vi "EXAMPLE_2.vi"() -> ()   [LabVIEW 2017]
uses:
  ZBOX_IS.lvlib
  <vilib>/Analysis/NI_AALBase.lvlib
  <vilib>/Analysis/baseanly.llb/Mean (DBL).vi
panel:
  in  "Get configuration data":bool
  in  "load comp":bool
  in  "load shunt":bool
  in  "Device Configuration File":path=path "SELECT Device Configuration File"
  out "Level":T1={"Slide 5"={1482, 2181}, "max OL 10"=FALSE, "max OL 9"=FALSE, "Slide 4"={1477, 2189}, "max OL 8"=FALSE, "max OL 7"=FALSE} {"Slide 4" scale=0.0..4096.0; "Slide 5" scale=0.0..4096.0}
  out "Application":string="EXAMPLE_3_1.vi"
  out "Battery Status":dbl
  out "Battery Voltage":dbl
  in  "DATA STREAMING":bool=TRUE
  out "writing":bool
  in  "Datalog file":string="Datalog_file_1.txt"
  out "CompValues":string="1000000000.00,1000000000.00,1000000000.00,1000000000.00,1000000000.00,1000000000.00,1000000000.00,1000000000.00,1000000000.00,1000000000.00,1000000000.00,1000000000.00,1000000000.00,1000000000.00,1000000000.00,       0.00,       0.00,       0.00,       0.00,       0.00,       0.00,       0.00,       0.00,       0.00,       0.00,       0.00,       0.00,       0.00,       0.00,       0.00"
  out "Shunt":string="     999.93,     999.93,     999.93,     999.93,     999.93,     999.93,     999.93,     999.93,     999.93,     999.93,     999.93,     999.93,     999.93,     999.92,     999.91,      -0.02,      -0.03,      -0.05,      -0.11,      -0.17,      -0.26,      -0.35,      -0.47,      -0.65,      -0.92,      -1.34,      -1.91,      -2.70,      -3.78,      -5.26"
  out "Frequencies":string="    1000.00Hz,    2000.00Hz,    3000.00Hz,    7000.00Hz,   11000.00Hz,   17000.00Hz,   23000.00Hz,   31000.00Hz,   43000.00Hz,   61000.00Hz,   89000.00Hz,  127000.00Hz,  179000.00Hz,  251000.00Hz,  349000.00Hz"
  in  "SAVE":bool
  out "Front End":string
  out "frequencies":dbl[](array[numeric])=[1000.0, 2000.0, 3000.0, 7000.0, 11000.0, 17000.0, 23000.0, 31000.0, 43000.0, 61000.0, 89000.0, 127000.0, 179000.0, 251000.0, 349000.0]
  out "DEVICE":bool
  out "Device":string
  in  "Ext_Trigger":bool
  in  "EN COMP":bool
  in  "MEAS COMP":bool
  in  "G2":u8(slide) scale=0.0..3.0
  in  "G1":u8(slide) scale=0.0..3.0
  out "Magnitude,   ohm":cluster{"freqs":dbl[], dbl[]}(graph)={"freqs"=[1000.0, 2000.0, 3000.0, 7000.0, 11000.0, 17000.0, 23000.0, 31000.0, 43000.0, 61000.0, 89000.0, 127000.0, 179000.0, 251000.0, 349000.0], [996.1091027832031, 996.1116979980469, 996.0496057128906, 996.1361779785157, 996.0625866699219, 996.056845703125, 996.0880285644531, 996.0972033691406, 996.0096704101562, 996.0107141113281, 995.8494006347656, 995.4951928710938, 994.7552624511719, 993.43984375, 991.5672961425781]}
  out "Phase, deg":cluster{"freqs":dbl[], dbl[]}(graph)={"freqs"=[1000.0, 2000.0, 3000.0, 7000.0, 11000.0, 17000.0, 23000.0, 31000.0, 43000.0, 61000.0, 89000.0, 127000.0, 179000.0, 251000.0, 349000.0], [-0.002247831257991493, -0.002652753913716879, -0.005691929007298313, -0.012889227512059733, -0.021220838949084282, -0.02892146535217762, -0.03975417457520962, -0.055281588807702065, -0.07622284047305584, -0.10836573675274849, -0.1603422838449478, -0.22576678663492203, -0.3038424688577652, -0.3925769108533859, -0.4546267157793045]}
  out "Connected":bool
  out "DFTBins":u16[](array[numeric])=[1, 2, 3, 7, 11, 17, 23, 31, 43, 61, 89, 127, 179, 251, 349]
  out "Status":string
  in  "Power Source":bool
  in  "Signal":u32(slide)=46 scale=0.0..100.0
  in  "Sample Rate Divider":u32(ring)=1 items=["1"=1, "2"=2, "4"=4, "6"=6, "8"=8, "10"=10, "12"=12, "14"=14, "16"=16, "20"=20, "24"=24, "28"=28, "32"=32, "40"=40, "48"=48, "56"=56, "64"=64, "80"=80, "96"=96, "112"=112, "128"=128, "160"=160, "192"=192, "196"=196, "224"=224, "256"=256, "320"=320, "384"=384, "448"=448, "512"=512, "640"=640, "768"=768, "896"=896, "1024"=1024, "1280"=1280, "1536"=1536, "1792"=1792]
  in  "stop":bool
  in  "# of packages":u32=50 min=1 step=1
  # "10"
  # "5"
  # "2"
  # "1"
  # "10"
  # "5"
  # "2"
  # "1"
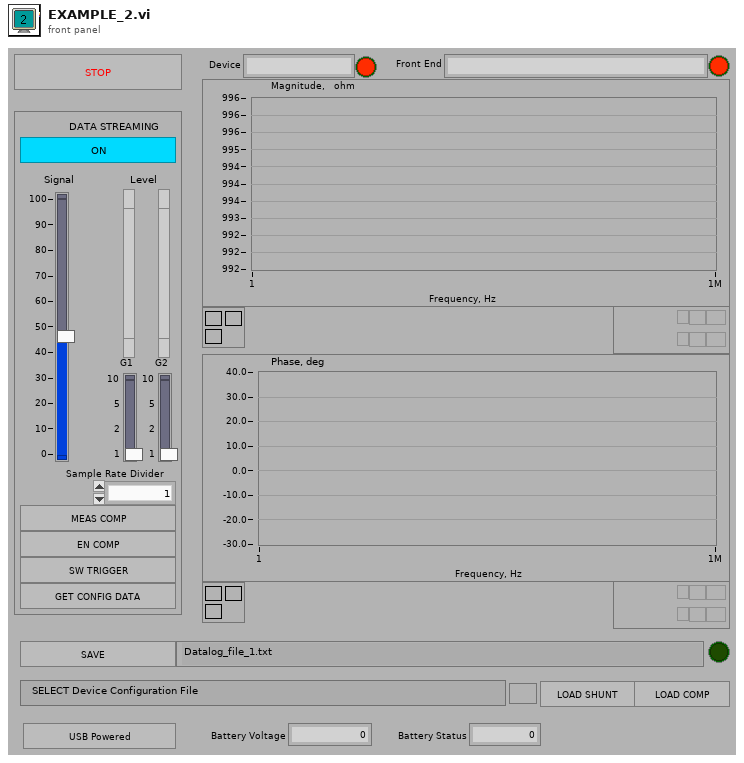
[diagram p1: front panel]
types:
  T1 = cluster{"Slide 5":cluster{u16, u16}, "max OL 10":bool, "max OL 9":bool, "Slide 4":cluster{u16, u16}, "max OL 8":bool, "max OL 7":bool}
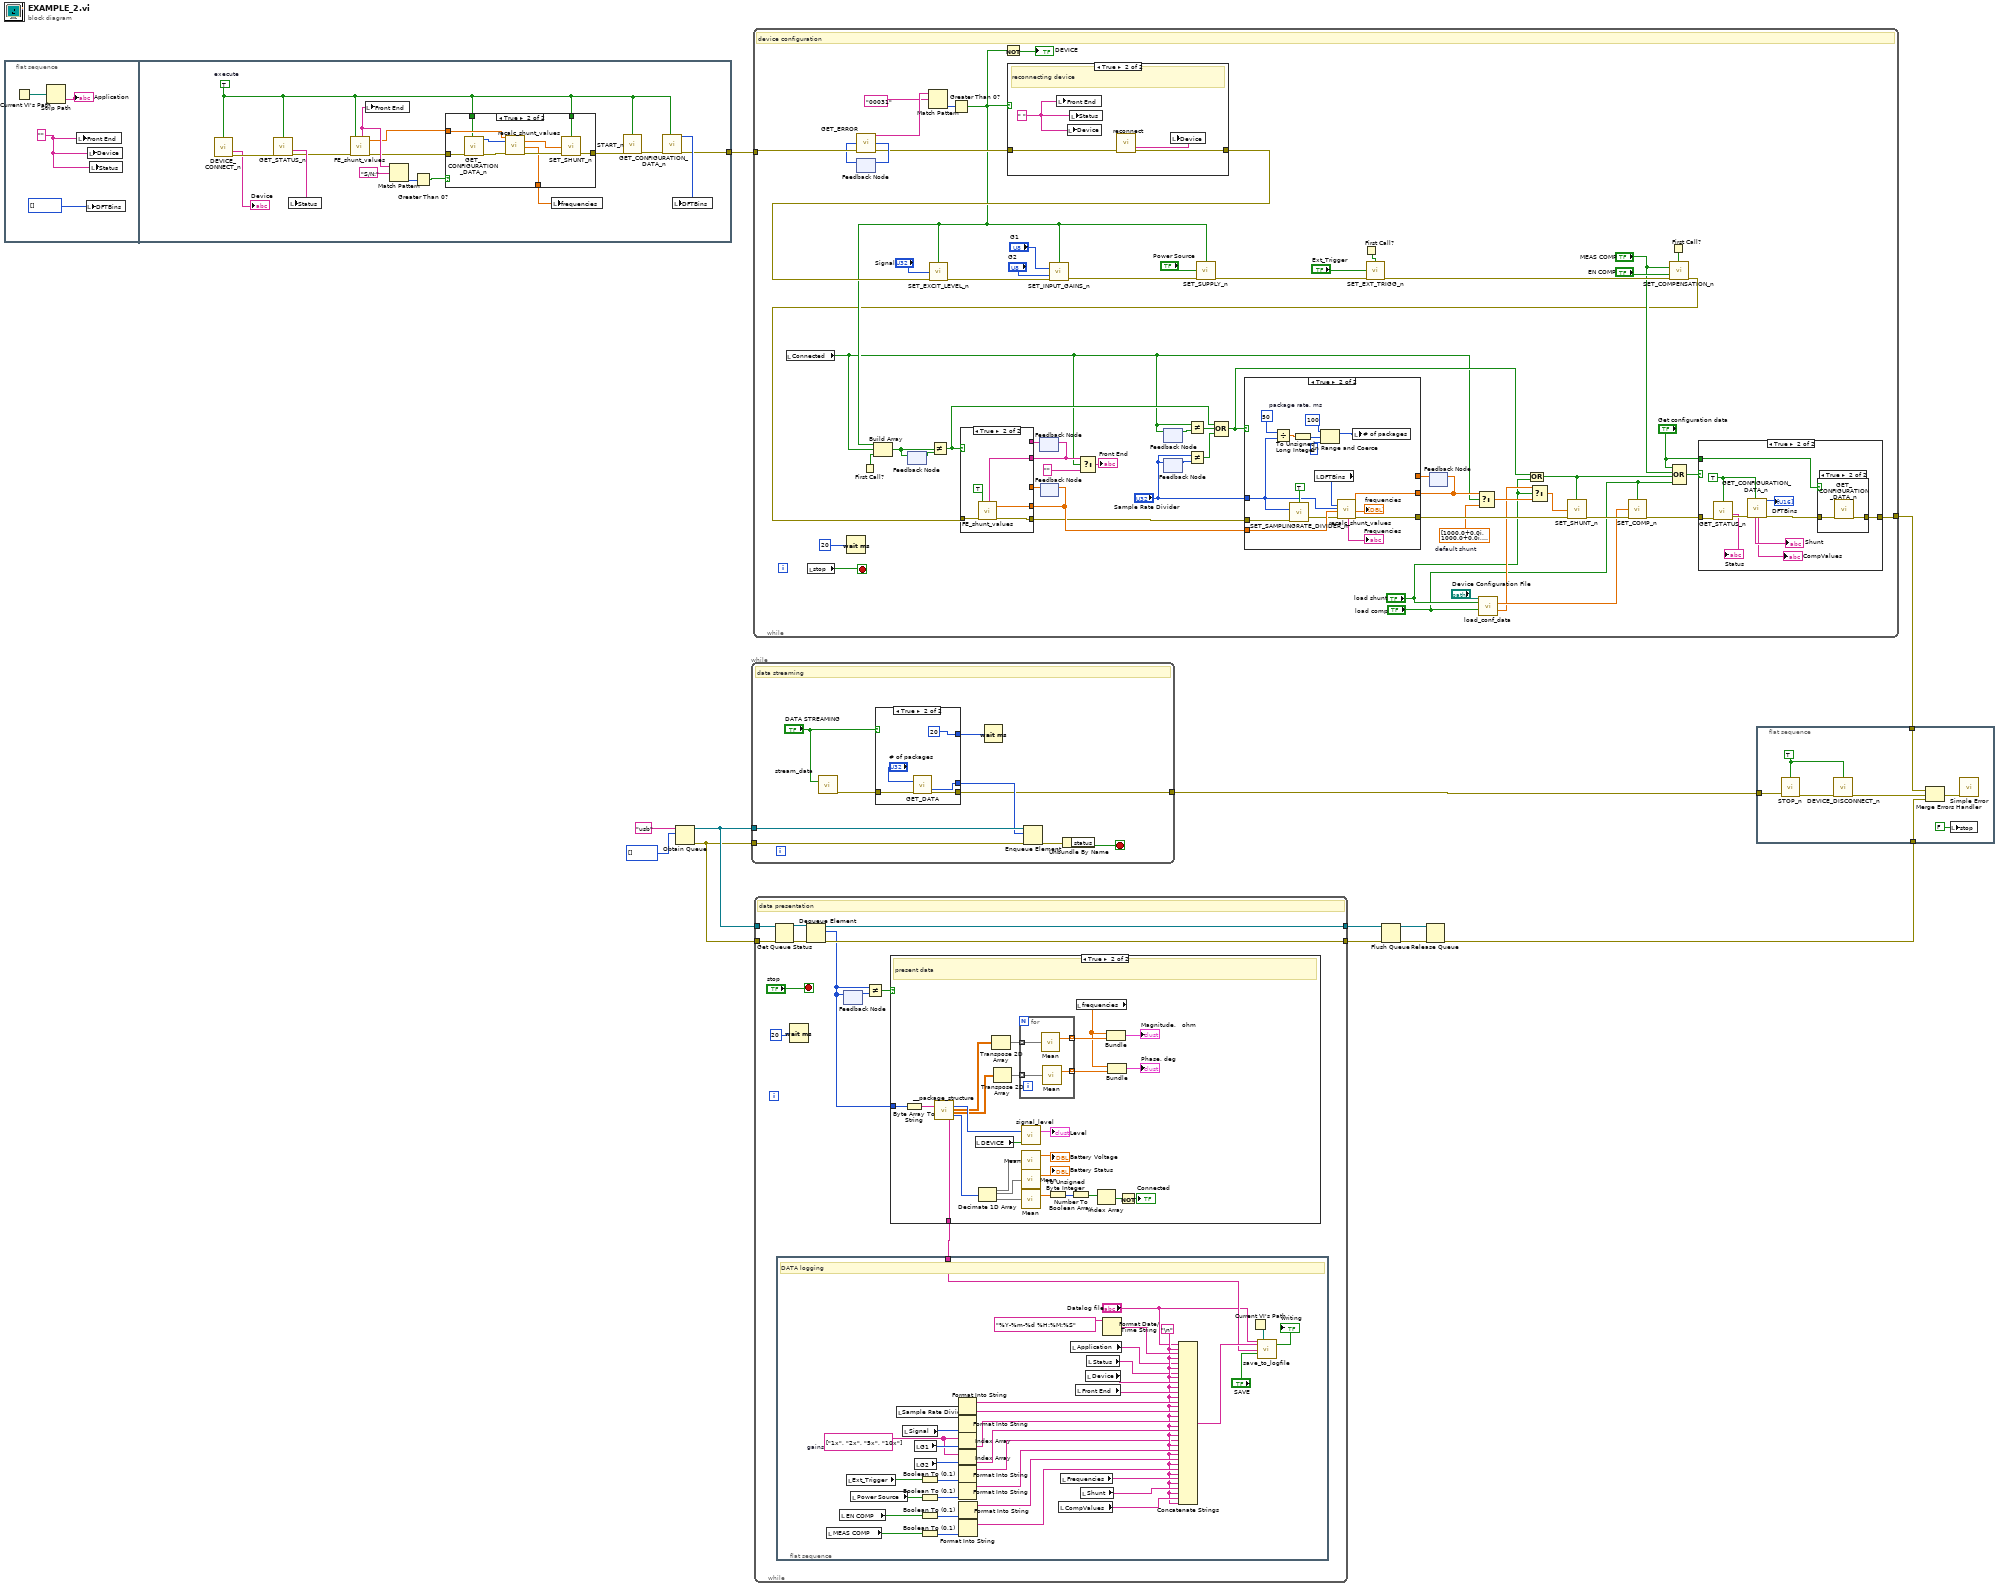
[diagram p0: block diagram]
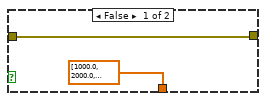
[diagram p2: hidden frame]
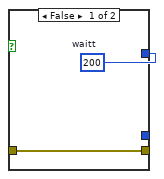
[diagram p3: hidden frame]
diagram:
  n1 = flat-sequence {
    tunnel: [w18] -> w7
    frame #0 {
      w16 = "" ("function return 2")
      n2 = Current VI's Path() -> (path=w13:path)
      n3 = Strip Path(path=w13) -> (name=→"Application":string)  [unwired: 1 out]
      n4 = local write "Front End"(w16) -> ()
      n5 = local write "DFTBins"(i32[] [] ("DFTBins")) -> ()
      n6 = local write "Device"(w16) -> ()
      n7 = local write "Status"(w16) -> ()
    }
    frame #1 {
      w17 = TRUE  # execute
      n8 = call "DEVICE_CONNECT_n.vi"("execute"=w17) -> ("serial no"=→"Device":string, "error out"=w32:errorcluster)  [unwired: 11 in, 2 out]
      n9 = call "GET_STATUS_n.vi"("execute"=w17, "error in (no error)"=w32) -> ("serial no"=w30:string, "error out"=w22:errorcluster)  [unwired: 10 in, 2 out]
      n10 = local write "Status"(w30) -> ()
      n11 = call "FE_shunt_values.vi"("error in (no error)"=w22, "execute"=w17) -> ("shunt"=w28:string, "FE_shunt_data"=w23:sgl[], "error out"=w24:errorcluster)  [unwired: 14 in, 1 out]
      n12 = local write "Front End"(w28) -> ()
      n13 = Match Pattern(string=w28, regular expression="S/N:") -> (offset past match=w26:i32)  [unwired: 1 in, 3 out]
      n14 = Greater Than 0?(x=w26) -> (x > 0?=w29:bool)
      n15 = case shown="True" w29 {
        tunnel: w23 -> [_ w44]
        tunnel: w24 -> [w33 w41]
        tunnel: [dbl[] [1000.0, 2000.0, 3000.0, 7000.0, 11000.0, 17000.0, 23000.0, 31000.0, 43000.0, 61000.0, 89000.0, 127000.0, 179000.0, 251000.0, 349000.0] ("freqs") w38] -> w25
        tunnel: [w33 w37] -> w21
        tunnel: w17 -> [_ w36]
        tunnel: w17 -> [_ w35]
        frame False {
        }
        frame True {
          n16 = call "GET_CONFIGURATION_DATA_n.vi"("error in (no error)"=w41, "execute"=w36) -> ("DFTBins"=w39:u16[], "error out"=w40:errorcluster)  [unwired: 7 in, 9 out]
          n17 = call "recalc_shunt_values.vi"("DFTBins"=w39, "FE_shunt_data"=w44, "error in (no error)"=w40) -> ("shunt"=w42:cdb[], "freqs"=w38:dbl[], "error out"=w43:errorcluster)  [unwired: 13 in, 1 out]
          n18 = call "SET_SHUNT_n.vi"("execute"=w35, "SHUNT values"=w42, "error in (no error)"=w43) -> ("error out"=w37:errorcluster)  [unwired: 11 in, 1 out]
        }
      }
      n19 = local write "frequencies"(w25) -> ()
      n20 = call "START_n.vi"("execute"=w17, "error in (no error)"=w21) -> ("error out"=w19:errorcluster)  [unwired: 12 in, 1 out]
      n21 = call "GET_CONFIGURATION_DATA_n.vi"("error in (no error)"=w19, "execute"=w17) -> ("DFTBins"=w20:u16[], "error out"=w18:errorcluster)  [unwired: 7 in, 9 out]
      n22 = local write "DFTBins"(w20) -> ()
    }
  }
  n23 = Obtain Queue(name (unnamed)="usb", element data type=u8[] [] ("unsigned byte array 2")) -> (queue out=w9:refnum<queue>, error out=w8:errorcluster)  [unwired: 3 in, 1 out]
  n24 = while {
    tunnel: w9 -> [w53]
    tunnel: w8 -> [w52]
    tunnel: [w46] -> w6
    stop <- w51 stop-if-true
    # "data streaming"
    n25 = call "stream_data.vi"("DATA STREAMING"="DATA STREAMING") -> ("error out"=w49:errorcluster)  [unwired: 14 in]
    n26 = case shown="True" "DATA STREAMING" {
      tunnel: [_ w60] -> w47
      tunnel: [w54 u32 20 ("wait")] -> w50
      tunnel: w49 -> [w55 w59]
      tunnel: [w55 w58] -> w46
      frame False {
        w54 = u32 200  # waitt
      }
      frame True {
        n27 = call "GET_DATA.vi"("ulValue"="# of packages", "error in (no error)"=w59) -> ("BytePtr"=w60:u8[], "error out"=w58:errorcluster)  [unwired: 11 in, 1 out]
      }
    }
    n28 = Wait (ms)(milliseconds to wait=w50) -> ()  [unwired: 1 out]
    n29 = Enqueue Element(queue=w53, element=w47, error in (no error)=w52) -> (error out=w45:errorcluster)  [unwired: 3 out]
    n30 = Unbundle By Name(w45) -> ("status"=w51:bool)
  }
  n31 = while {
    tunnel: w7 -> [w109]
    tunnel: [w71] -> w4
    stop <- w61 stop-if-true
    w94 = cdb[] [1000.0+0.0i, 1000.0+0.0i, 1000.0+0.0i, 1000.0+0.0i, 1000.0+0.0i, 1000.0+0.0i, 1000.0+0.0i, 1000.0+0.0i, 1000.0+0.0i, 1000.0+0.0i, 1000.0+0.0i, 1000.0+0.0i, 1000.0+0.0i, 1000.0+0.0i, 1000.0+0.0i]  # default shunt
    # "device configuration"
    n32 = local read "Connected"() -> (w78:bool)
    n33 = local read "stop"() -> (w61:bool)
    n34 = Wait (ms)(milliseconds to wait=u32 20 ("wait")) -> ()  [unwired: 1 out]
    n35 = feedback #1() -> (w106:u32[])  [unwired: 1 in]
    n36 = call "GET_ERROR.vi"("uLPtr"=w106, "error in (no error)"=w109) -> ("function return"=w105:string, "uLPtr"=w107:u32[], "error out"=w103:errorcluster)  [unwired: 11 in]
    n37 = feedback-in #1(w107) -> ()
    n38 = First Call?() -> (First Call?: T/F=w98:bool)
    n39 = feedback #2() -> (w93:bool[])  [unwired: 1 in]
    n40 = Match Pattern(string=w105, regular expression="00031" ("substring 2")) -> (offset past match=w108:i32)  [unwired: 1 in, 3 out]
    n41 = Greater Than 0?(x=w108) -> (x > 0?=w83:bool)
    n42 = Build Array(w83, w78, w98) -> (w92:bool[])
    n43 = feedback-in #2(w92) -> ()
    n44 = Not Equal?(x=w92, y=w93) -> (x != y?=w79:bool)
    n45 = Not(x=w83) -> (.not. x?=→"DEVICE":bool)
    n46 = case shown="True" w83 {
      tunnel: w103 -> [w122 w126]
      tunnel: [w122 w125] -> w97
      frame False {
      }
      frame True {
        w123 = " " ("status")
        # "reconnecting device"
        n47 = local write "Front End"(w123) -> ()
        n48 = local write "Device"(w123) -> ()
        n49 = local write "Status"(w123) -> ()
        n50 = call "reconnect.vi"("error in (no error)"=w126) -> ("serial no"=w124:string, "error out"=w125:errorcluster)  [unwired: 12 in, 1 out]
        n51 = local write "Device"(w124) -> ()
      }
    }
    n52 = call "SET_EXCIT_LEVEL_n.vi"("execute"=w83, "Level"="Signal", "error in (no error)"=w97) -> ("error out"=w117:errorcluster)  [unwired: 11 in, 1 out]
    n53 = feedback #3() -> (w115:string)  [unwired: 1 in]
    n54 = feedback #4() -> (w116:sgl[])  [unwired: 1 in]
    n55 = call "SET_INPUT_GAINS_n.vi"("execute"=w83, "G1"="G1", "G2"="G2", "error in (no error)"=w117) -> ("error out"=w110:errorcluster)  [unwired: 10 in, 1 out]
    n56 = feedback #5() -> (w91:bool)  [unwired: 1 in]
    n57 = feedback-in #5(w78) -> ()
    n58 = feedback #6() -> (w90:u32)  [unwired: 1 in]
    n59 = feedback-in #6("Sample Rate Divider") -> ()
    n60 = Not Equal?(x=w78, y=w91) -> (x != y?=w82:bool)
    n61 = Not Equal?(x="Sample Rate Divider", y=w90) -> (x != y?=w80:bool)
    n62 = call "SET_SUPPLY_n.vi"("execute"=w83, "supply"="Power Source", "error in (no error)"=w110) -> ("error out"=w73:errorcluster)  [unwired: 11 in, 1 out]
    n63 = Compound Arithmetic op=OR(w79, w82, w80) -> (w81:bool)
    n64 = First Call?() -> (First Call?: T/F=w75:bool)
    n65 = call "SET_EXT_TRIGG_n.vi"("execute"=w75, "EXT_TRIGG"="Ext_Trigger", "error in (no error)"=w73) -> ("error out"=w72:errorcluster)  [unwired: 11 in, 1 out]
    n66 = feedback #7() -> (w114:cdb[])  [unwired: 1 in]
    n67 = call "load_conf_data.vi"("file"="Device Configuration File", "SET Shunt"="load shunt", "SET Compensation"="load comp") -> ("Comp"=w67:cdb[], "Shunt"=w66:cdb[])  [unwired: 11 in]
    n68 = Or(x=w81, y="load shunt") -> (x .or. y?=w70:bool)
    n69 = First Call?() -> (First Call?: T/F=w74:bool)
    n70 = call "SET_COMPENSATION_n.vi"("execute"=w74, "measure COMP value"="MEAS COMP", "COMPENSATION"="EN COMP", "error in (no error)"=w72) -> ("error out"=w62:errorcluster)  [unwired: 10 in, 1 out]
    n71 = case shown="True" w79 {
      tunnel: w62 -> [w143 w148]
      tunnel: [w143 w147] -> w99
      tunnel: [w142 w146] -> w100
      tunnel: w116 -> [w142 _]
      tunnel: [w141 w145] -> w96
      tunnel: w115 -> [w141 _]
      frame False {
      }
      frame True {
        n72 = call "FE_shunt_values.vi"("error in (no error)"=w148, "execute"=TRUE) -> ("shunt"=w145:string, "FE_shunt_data"=w146:sgl[], "error out"=w147:errorcluster)  [unwired: 14 in, 1 out]
      }
    }
    n73 = feedback-in #3(w96) -> ()
    n74 = feedback-in #4(w100) -> ()
    n75 = Select(t=w96, s=w78, f="" ("t")) -> (s? t:f=→"Front End":string)
    n76 = case shown="True" w81 {
      tunnel: "Sample Rate Divider" -> [_ w151]
      tunnel: w99 -> [w150 w154]
      tunnel: [w150 w159] -> w112
      tunnel: w100 -> [_ w157]
      tunnel: [w149 w155] -> w85
      tunnel: w114 -> [w149 _]
      frame False {
      }
      frame True {
        w166 = u32 50  # package rate, ms
        n77 = Divide(x=w166, y=w151) -> (x/y=w163:dbl)
        n78 = call "SET_SAMPLINGRATE_DIVIDER_n.vi"("execute"=TRUE, "ulValue"=w151, "error in (no error)"=w154) -> ("error out"=w153:errorcluster)  [unwired: 11 in, 1 out]
        n79 = To Unsigned Long Integer(number=w163) -> (unsigned 32bit integer=w164:u32)
        n80 = local read "DFTBins"() -> (w160:u16[])
        n81 = In Range and Coerce(upper limit=u32 100, x=w164, lower limit=u32 1) -> (coerced(x)=w161:u32)  [unwired: 1 out]
        n82 = call "recalc_shunt_values.vi"("DFTBins"=w160, "DIV"=w151, "FE_shunt_data"=w157, "error in (no error)"=w153) -> ("Frequencies"=→"Frequencies":string, "shunt"=w155:cdb[], "freqs"=→"frequencies":dbl[], "error out"=w159:errorcluster)  [unwired: 12 in]
        n83 = local write "# of packages"(w161) -> ()
      }
    }
    n84 = feedback-in #7(w85) -> ()
    n85 = Select(t=w85, s=w78, f=w94) -> (s? t:f=w84:cdb[])
    n86 = Select(t=w66, s="load shunt", f=w84) -> (s? t:f=w86:cdb[])
    n87 = call "SET_SHUNT_n.vi"("execute"=w70, "SHUNT values"=w86, "error in (no error)"=w112) -> ("error out"=w88:errorcluster)  [unwired: 11 in, 1 out]
    n88 = call "SET_COMP_n.vi"("execute"="load comp", "COMP values"=w67, "error in (no error)"=w88) -> ("error out"=w87:errorcluster)  [unwired: 11 in, 1 out]
    n89 = Compound Arithmetic op=OR("Get configuration data", "MEAS COMP", w70, "load comp") -> (w113:bool)
    n90 = case shown="True" w113 {
      tunnel: w87 -> [w127 w130]
      tunnel: [w127 w132] -> w71
      tunnel: "Get configuration data" -> [_ w134]
      frame False {
      }
      frame True {
        w129 = TRUE ("execute")
        n91 = call "GET_STATUS_n.vi"("execute"=w129, "error in (no error)"=w130) -> ("serial no"=→"Status":string, "error out"=w131:errorcluster)  [unwired: 10 in, 2 out]
        n92 = call "GET_CONFIGURATION_DATA_n.vi"("error in (no error)"=w131, "execute"=w129) -> ("Shunt"=→"Shunt":string, "CompValues"=→"CompValues":string, "DFTBins"=→"DFTBins":u16[], "error out"=w133:errorcluster)  [unwired: 7 in, 7 out]
        n93 = case shown="True" w134 {
          tunnel: w133 -> [w138 w140]
          tunnel: [w138 w139] -> w132
          frame False {
          }
          frame True {
            n94 = call "GET_CONFIGURATION_DATA_n.vi"("error in (no error)"=w140) -> ("error out"=w139:errorcluster)  [unwired: 10 in]
          }
        }
      }
    }
  }
  n95 = while {
    tunnel: w9 -> [w174]
    tunnel: w8 -> [w173]
    tunnel: [w171] -> w3
    tunnel: [w170] -> w2
    stop <- "stop" stop-if-true
    # "data presentation"
    n96 = Get Queue Status(queue=w174, error in (no error)=w173) -> (queue out=w177:refnum<queue>, error out=w176:errorcluster)  [unwired: 7 out]
    n97 = flat-sequence {
      tunnel: w172 -> [w184]
      frame #0 {
        w202 = string[] ["1x", "2x", "5x", "10x"]  # gains
        w188 = "\n"
        # "DATA logging"
        n98 = local read "MEAS COMP"() -> (w192:bool)
        n99 = local read "EN COMP"() -> (w193:bool)
        n100 = local read "Ext_Trigger"() -> (w207:bool)
        n101 = local read "Power Source"() -> (w204:bool)
        n102 = local read "Sample Rate Divider"() -> (w211:u32)
        n103 = local read "Signal"() -> (w209:u32)
        n104 = local read "G1"() -> (w203:u8)
        n105 = local read "G2"() -> (w201:u8)
        n106 = Boolean To (0,1)(Boolean=w207) -> (0, 1=w206:i16)
        n107 = Boolean To (0,1)(Boolean=w204) -> (0, 1=w205:i16)
        n108 = Boolean To (0,1)(Boolean=w193) -> (0, 1=w198:i16)
        n109 = Boolean To (0,1)(Boolean=w192) -> (0, 1=w195:i16)
        n110 = Format Into String(w211) -> (resulting string=w210:string)  [unwired: 3 in, 1 out]
        n111 = Format Into String(w209) -> (resulting string=w208:string)  [unwired: 3 in, 1 out]
        n112 = Index Array(array=w202, index=w203) -> (element=w200:string)
        n113 = Index Array(array=w202, index=w201) -> (element=w199:string)
        n114 = Format Into String(w206) -> (resulting string=w182:string)  [unwired: 3 in, 1 out]
        n115 = Format Into String(w205) -> (resulting string=w197:string)  [unwired: 3 in, 1 out]
        n116 = Format Into String(w198) -> (resulting string=w196:string)  [unwired: 3 in, 1 out]
        n117 = Format Into String(w195) -> (resulting string=w194:string)  [unwired: 3 in, 1 out]
        n118 = local read "CompValues"() -> (w189:string)
        n119 = local read "Frequencies"() -> (w191:string)
        n120 = local read "Application"() -> (w180:string)
        n121 = local read "Front End"() -> (w212:string)
        n122 = local read "Shunt"() -> (w190:string)
        n123 = local read "Device"() -> (w213:string)
        n124 = local read "Status"() -> (w181:string)
        n125 = Format Date/Time String(time format string (%c)="%Y-%m-%d %H:%M:%S") -> (date/time string=w215:string)  [unwired: 1 in, 1 out]
        n126 = Concatenate Strings("Datalog file", w188, w215, w188, w180, w188, w181, w188, w213, w188, w212, w188, w210, w188, w208, w188, w200, w188, w199, w188, w182, w188, w197, w188, w196, w188, w194, w188, w191, w188, w190, w188, w189, w188) -> (w186:string)
        n127 = Current VI's Path() -> (path=w183:path)
        n128 = call "save_to_logfile.vi"("file"="Datalog file", "header_data"=w186, "to logfile"=w184, "SAVE"="SAVE", "path"=w183) -> ("writing"=→"writing":bool)  [unwired: 13 in, 1 out]
      }
    }
    n129 = Wait (ms)(milliseconds to wait=u32 20 ("wait")) -> ()  [unwired: 1 out]
    n130 = Dequeue Element(queue=w177, error in (no error)=w176) -> (queue out=w171:refnum<queue>, element=w168:u8[], error out=w170:errorcluster)  [unwired: 1 in, 1 out]
    n131 = feedback #8() -> (w169:u8[])  [unwired: 1 in]
    n132 = feedback-in #8(w168) -> ()
    n133 = Not Equal?(x=w168, y=w169) -> (x != y?=w167:bool)
    n134 = case shown="True" w167 {
      tunnel: w168 -> [_ w241]
      tunnel: [_ w227] -> w172
      frame False {
      }
      frame True {
        # "present data"
        n135 = Byte Array To String(unsigned byte array=w241) -> (string=w236:string)
        n136 = call "__package_structure.vi"("data"=w236) -> ("to logfile"=w227:string[], "max_min"=w235:u16[], "M"=w217:sgl[][], "Ph"=w216:sgl[][], "status"=w234:u16[])  [unwired: 8 in, 6 out]
        n137 = local read "DEVICE"() -> (w221:bool)
        n138 = Decimate 1D Array(w234) -> (w225:u16[], w224:u16[], w233:u16[])
        n139 = Transpose 2D Array(2D array=w217) -> (transposed array=w240:sgl[][])
        n140 = Transpose 2D Array(2D array=w216) -> (transposed array=w239:sgl[][])
        n141 = for {
          tunnel: w240 -> [w245] mode=indexing
          tunnel: [w244] -> w238 mode=indexing
          tunnel: w239 -> [w242] mode=indexing
          tunnel: [w243] -> w237 mode=indexing
          n142 = call-poly <vilib>:"Mean.vi"("X"=w245) -> ("mean"=w244:dbl)  [unwired: 1 out]
          n143 = call-poly <vilib>:"Mean.vi"("X"=w242) -> ("mean"=w243:dbl)  [unwired: 1 out]
        }
        n144 = call-poly <vilib>:"Mean.vi"("X"=w225) -> ("mean"=→"Battery Voltage":dbl)  [unwired: 1 out]
        n145 = call-poly <vilib>:"Mean.vi"("X"=w224) -> ("mean"=→"Battery Status":dbl)  [unwired: 1 out]
        n146 = call-poly <vilib>:"Mean.vi"("X"=w233) -> ("mean"=w226:dbl)  [unwired: 1 out]
        n147 = call "signal_level.vi"("data U16"=w235, "signal?"=w221) -> ("level"=→"Level":T1)  [unwired: 13 in]
        n148 = To Unsigned Byte Integer(number=w226) -> (unsigned 8bit integer=w232:u8)
        n149 = Number To Boolean Array(number=w232) -> (Boolean array=w231:bool[])
        n150 = local read "frequencies"() -> (w230:dbl[])
        n151 = Index Array(array=w231) -> (element=w220:bool)  [unwired: 1 in]
        n152 = Bundle("frequencies"=w230, w238) -> (→"Magnitude,   ohm":cluster{"frequencies":dbl[], dbl[]})  [unwired: 1 in]
        n153 = Bundle("frequencies"=w230, w237) -> (→"Phase, deg":cluster{"frequencies":dbl[], dbl[]})  [unwired: 1 in]
        n154 = Not(x=w220) -> (.not. x?=→"Connected":bool)
      }
    }
  }
  n155 = Flush Queue(queue=w3, error in (no error)=w2) -> (queue out=w10:refnum<queue>, error out=w11:errorcluster)  [unwired: 1 out]
  n156 = Release Queue(queue=w10, error in (no error)=w11) -> (error out=w1:errorcluster)  [unwired: 3 out]
  n157 = flat-sequence {
    tunnel: w6 -> [w252]
    tunnel: w4 -> [w249]
    tunnel: w1 -> [w248]
    frame #0 {
      w247 = TRUE ("execute")
      n158 = call "STOP_n.vi"("execute"=w247, "error in (no error)"=w252) -> ("error out"=w253:errorcluster)  [unwired: 12 in, 1 out]
      n159 = call "DEVICE_DISCONNECT_n.vi"("execute"=w247, "error in (no error)"=w253) -> ("error out"=w251:errorcluster)  [unwired: 12 in, 1 out]
      n160 = Merge Errors(w249, w251, w248) -> (w250:errorcluster)
      n161 = local write "stop"(FALSE ("stop")) -> ()
      n162 = call <vilib>:"Simple Error Handler.vi"("error in (no error)"=w250) -> ()  [unwired: 4 in, 5 out]
    }
  }
